vi "Execute Show-Attached-Object--Menu-for-BD-Comments.vi"(6 "Mouse Position":T1, 8 "User VI Ref":refnum<vi>, 9 "Menu Item Tag Suffix":string, 10 "Remaining Items":refnum<vi>[](array[refnum]), 11 "Affected Items":T2) -> (0 "Fail transaction?":bool)   [LabVIEW 2020]
doc: "This VI is part of a plug-in for modifying the LabVIEW shortcut menus. This is the execute VI which is called when the shortcut menu is chosen by the user. It performs the action of the selected menu item."
uses:
  Show-Attached-Object--Menu-for-BD-Comments.ctl
  <vilib>/Utility/miscctls.llb/LVPositionTypeDef.ctl
panel:
  # "All controls on this panel except \"Affected Items\" have been locked to prevent accidental edits. Changing the control names or types, other than the elements of the \"Affected Items\" cluster will make the VI unusable as a menu plugin.\n\nSee Context Help for each control for details about its use."
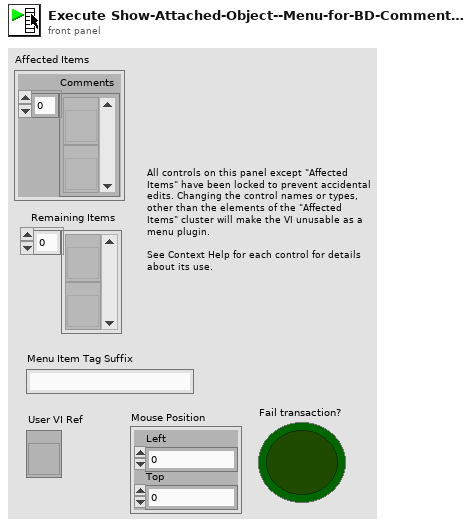
[diagram p1: front panel]
types:
  T1 = typedef "LVPositionTypeDef.ctl" = cluster{"Left":i32, "Top":i32}
  T2 = typedef "Show-Attached-Object--Menu-for-BD-Comments.ctl" = cluster{"Comments":refnum<vi>[]}
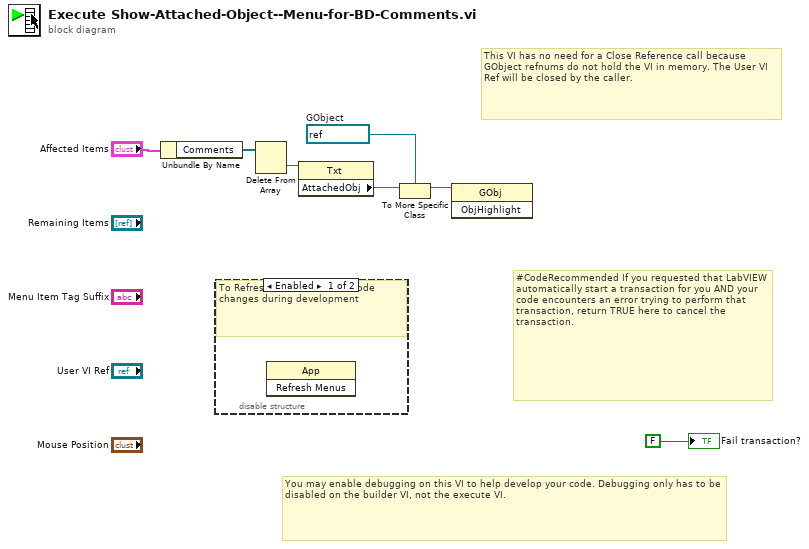
[diagram p0: block diagram]
diagram:
  w1 = refnum<vi> refnum  # GObject
  # "You may enable debugging on this VI to help develop your code. Debugging only has to be disabled on the builder VI, not the execute VI."
  # "#CodeRecommended If you requested that LabVIEW automatically start a transaction for you AND your code encounters an error trying to perform that transaction, return TRUE here to cancel the transaction."
  # "This VI has no need for a Close Reference call because GObject refnums do not hold the VI in memory. The User VI Ref will be closed by the caller."
  n1 = Unbundle By Name("Affected Items") -> ("Comments"=w4:refnum<vi>[])
  n2 = disable-structure shown="Enabled" {
    frame Enabled {
      # "To Refresh the Menus after code changes during development"
      n3 = invoke class="App" method="Refresh Menus"() -> ()  [unwired: 3 in, 3 out]
    }
    frame Disabled {
    }
  }
  n4 = Delete From Array(array=w4) -> (deleted portion=w5:refnum<vi>)  [unwired: 2 in, 1 out]
  n5 = property class="Txt"(reference=w5) -> ("AttachedObj"=w3:refnum<vi>)  [unwired: 1 in, 2 out]
  n6 = To More Specific Class(target class=w1, reference=w3) -> (specific class reference=w2:refnum<vi>)  [unwired: 1 in, 1 out]
  n7 = invoke class="GObj" method="ObjHighlight"(reference=w2) -> ()  [unwired: 2 in, 3 out]
  "Fail transaction?" <- FALSE ("Fail transaction?")
